vi "Check Green and Red LEDs.vi"(8 "error in":errorcluster, 9 "Voltage On Red":dbl, 10 "Voltage On Green":dbl, 11 "DMM":refnum<visa-resource-name>="COM1") -> (0 "error out":errorcluster, 1 "LED Voltages":dbl[](array[numeric]), 2 "Voltage Red":dbl format="%0.2f", 3 "Voltage Green":dbl format="%0.2f", 4 "D4 Red OFF":bool, 5 "D4 Green Off":bool, 6 "D4 Red On":bool, 7 "D4 Green On":bool)   [LabVIEW 2015]
uses:
  <instrlib>/Keithley 27XX/Keithley 27XX.lvlib
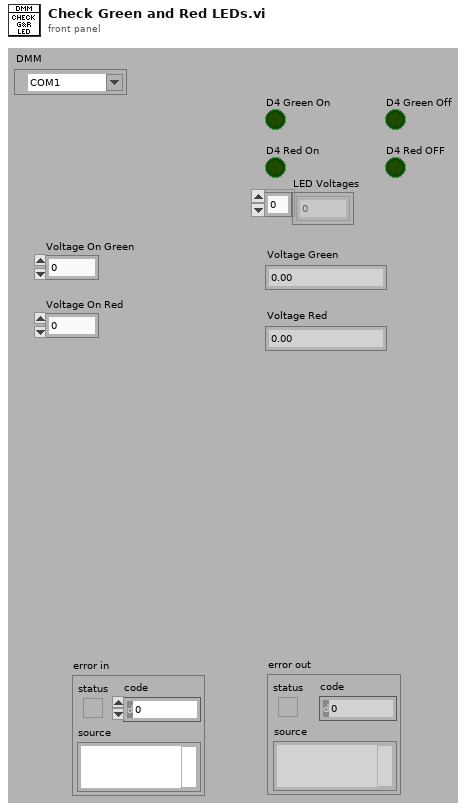
[diagram p1: front panel]
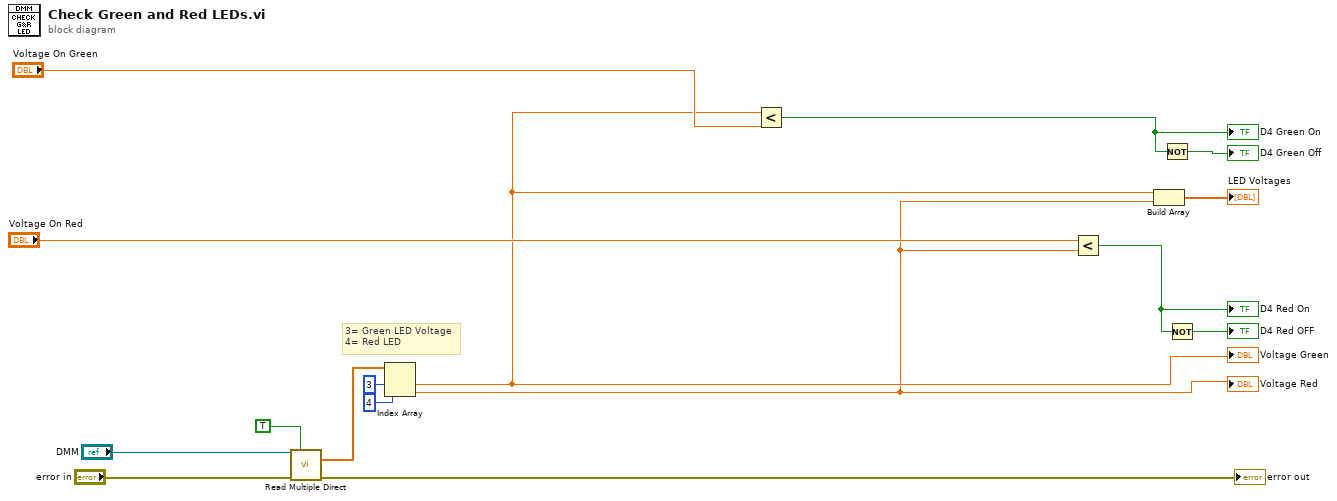
[diagram p0: block diagram]
diagram:
  # "3= Green LED Voltage\n4= Red LED"
  n1 = call <instrlib>:"Read Multiple Direct.vi"("VISA resource name"="DMM", "All Data Elements (False)"=TRUE, "error in (no error)"="error in") -> ("Measurement Data"=w3:dbl[], "error out"=→"error out":errorcluster)  [unwired: 7 in, 4 out]
  n2 = Index Array(array=w3, index #1=3 ("index"), index #2=4 ("index")) -> (element #1=w8:dbl, element #2=w7:dbl)
  "Voltage Red" <- w7
  "Voltage Green" <- w8
  n3 = Less?(x=w8, y="Voltage On Green") -> (x < y?=w11:bool)
  "D4 Green On" <- w11
  n4 = Less?(x="Voltage On Red", y=w7) -> (x < y?=w10:bool)
  "D4 Red On" <- w10
  n5 = Build Array(w8, w7) -> (→"LED Voltages":dbl[])
  n6 = Not(x=w11) -> (.not. x?=→"D4 Green Off":bool)
  n7 = Not(x=w10) -> (.not. x?=→"D4 Red OFF":bool)
